vi "LauncherSpeedByDistance.vi"() -> (3 "output speed":dbl)   [LabVIEW 2015]
uses:
  Distance.vi
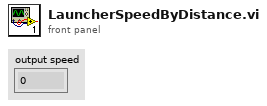
[diagram p1: front panel]
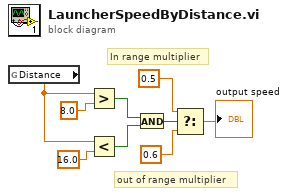
[diagram p0: block diagram]
diagram:
  # "out of range multiplier"
  # "In range multiplier"
  n1 = global read "Distance.vi" "Distance"() -> (w8:dbl)
  n2 = Greater?(x=w8, y=8.0) -> (0:w9:bool)
  n3 = Less?(x=w8, y=16.0) -> (x < y?=w6:bool)
  n4 = And(x=w9, y=w6) -> (x .and. y?=w4:bool)
  n5 = Select(t=0.5, s=w4, f=0.6) -> (s? t:f=→"output speed":dbl)
